vi "MyFPGACode 2.vi"() -> ()   [LabVIEW 2013]
uses:
  <vilib>/Platform/TimedLoop/XDataNode/wakeup.ctl
  <vilib>/Platform/TimedLoop/XDataNode/XDNodeRunTimeDep.lvlib
  <vilib>/Platform/TimedLoop/XDataNode/nitl_modes.ctl
  <vilib>/Platform/TimedLoop/XDataNode/timing_clust.ctl
  <vilib>/Platform/TimedLoop/XDataNode/XDataNode.xnode
  <vilib>/eio/EIONode/EIONode.xnode
  <vilib>/rvi/eio/common/nirviEmuTemplateMethod_errors.vi
  <vilib>/rvi/Analysis/measure/butterworth/XNode/niFpgaButterworthFilter.xnode
  <vilib>/rvi/Analysis/measure/LMRsmpl/XNode/niFPGA Rational Resampler.xnode
  <vilib>/rvi/LocalResourceManager/LocalResourceManager.xnode
  <vilib>/rvi/DataTransferAndStorage/Container/XNode/niFpgaContainer.xnode
  <vilib>/rvi/FIFO/Fifo_Resource/niFpgaFifoEmulationRefIn.vi
  <vilib>/rvi/Analysis/common/codeGenErrors/XNode/niFpgaXNodeCodeGenErrorHandle.vi
  <vilib>/rvi/DataTransferAndStorage/Container/Common/niFpgaContainerGetUniqueNameForEmu.vi
  <vilib>/rvi/DataTransferAndStorage/Container/Common/niFpgaContainerSetEmuInfo.vi
  <vilib>/rvi/eio/common/nirviEmuReportErrorAndStop.vi
panel:
  in  "Start 0":bool
  in  "Filter On":bool=TRUE
  in  "Beta":fxp<+/-,24,0>
  out "Output 8":i16
  out "Output 7":i16
  out "Output 6":i16
  out "Output 5":i16
  out "Output 4":i16
  out "Output 3":i16
  out "Output 2":i16
  out "Output 1":i16
  out "Output 0":i16
  out "Input 8":i16
  out "Input 7":i16
  out "Input 6":i16
  out "Input 5":i16
  out "Input 4":i16
  out "Input 3":i16
  out "Input 2":i16
  out "Input 1":i16
  in  "Local Stop 0":bool
  out "Actual Loop Rate (Ticks)":u32
  out "Late? Latched":bool
  out "Input 0":i16
  in  "Loop Rate (Ticks)":u32=4000
  in  "Reset":bool
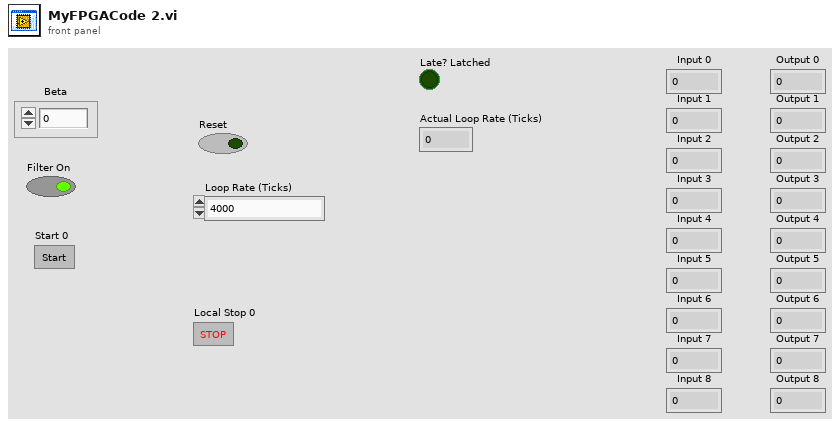
[diagram p1: front panel]
types:
  T1 = typedef "XDNodeRunTimeDep.lvlib/timing_clust.ctl" = cluster{"Expected End [f-1]":u64, "Actual End [f-1]":u64, "Finished Late? [f-1]":bool, "Expected End [i-1]":u64, "Actual End [i-1]":u64, "Finished Late? [i-1]":bool, "Expected Start [i]":u64, "Actual Start [i]":u64, "Expected Start [f]":u64, "Actual Start [f]":u64, "Source Name":string, "Structure Name":string, "Period":i64, "Deadline":i64, "Offset":i64, "Start":i64, "Priority":i32, "Timeout":i32, "Mode":T2, "Wakeup Reason":T3, "Error":errorcluster, "Source Type":string, "Secondary Source Type":string, "Global End Time":u64, "Global Start Time":u64, "Frame Duration":u64, "Iteration Duration":u64, "Assigned CPU":i32, "I/O Scan Engine Mode":u32}
  T2 = typedef "XDNodeRunTimeDep.lvlib/nitl_modes.ctl" = enum32{"No Change", "Process missed periods, maintain original phase", "Discard missed periods, maintain original phase", "Process missed periods, ignore original phase", "Discard missed periods, ignore original phase"}
  T3 = typedef "XDNodeRunTimeDep.lvlib/wakeup.ctl" = enum32{"Normal", "Aborted", "Asynchronous wakeup", "Timing source error", "Timed loop error", "Timeout"}
  T4 = cluster{"X":fxp<+/-,16,2>, "Y":fxp<+/-,16,2>, "Z":fxp<+/-,16,2>}
  T5 = cluster{"[0]":fxp<+/-,16,2>, "[1]":fxp<+/-,16,2>, "[2]":fxp<+/-,16,2>}
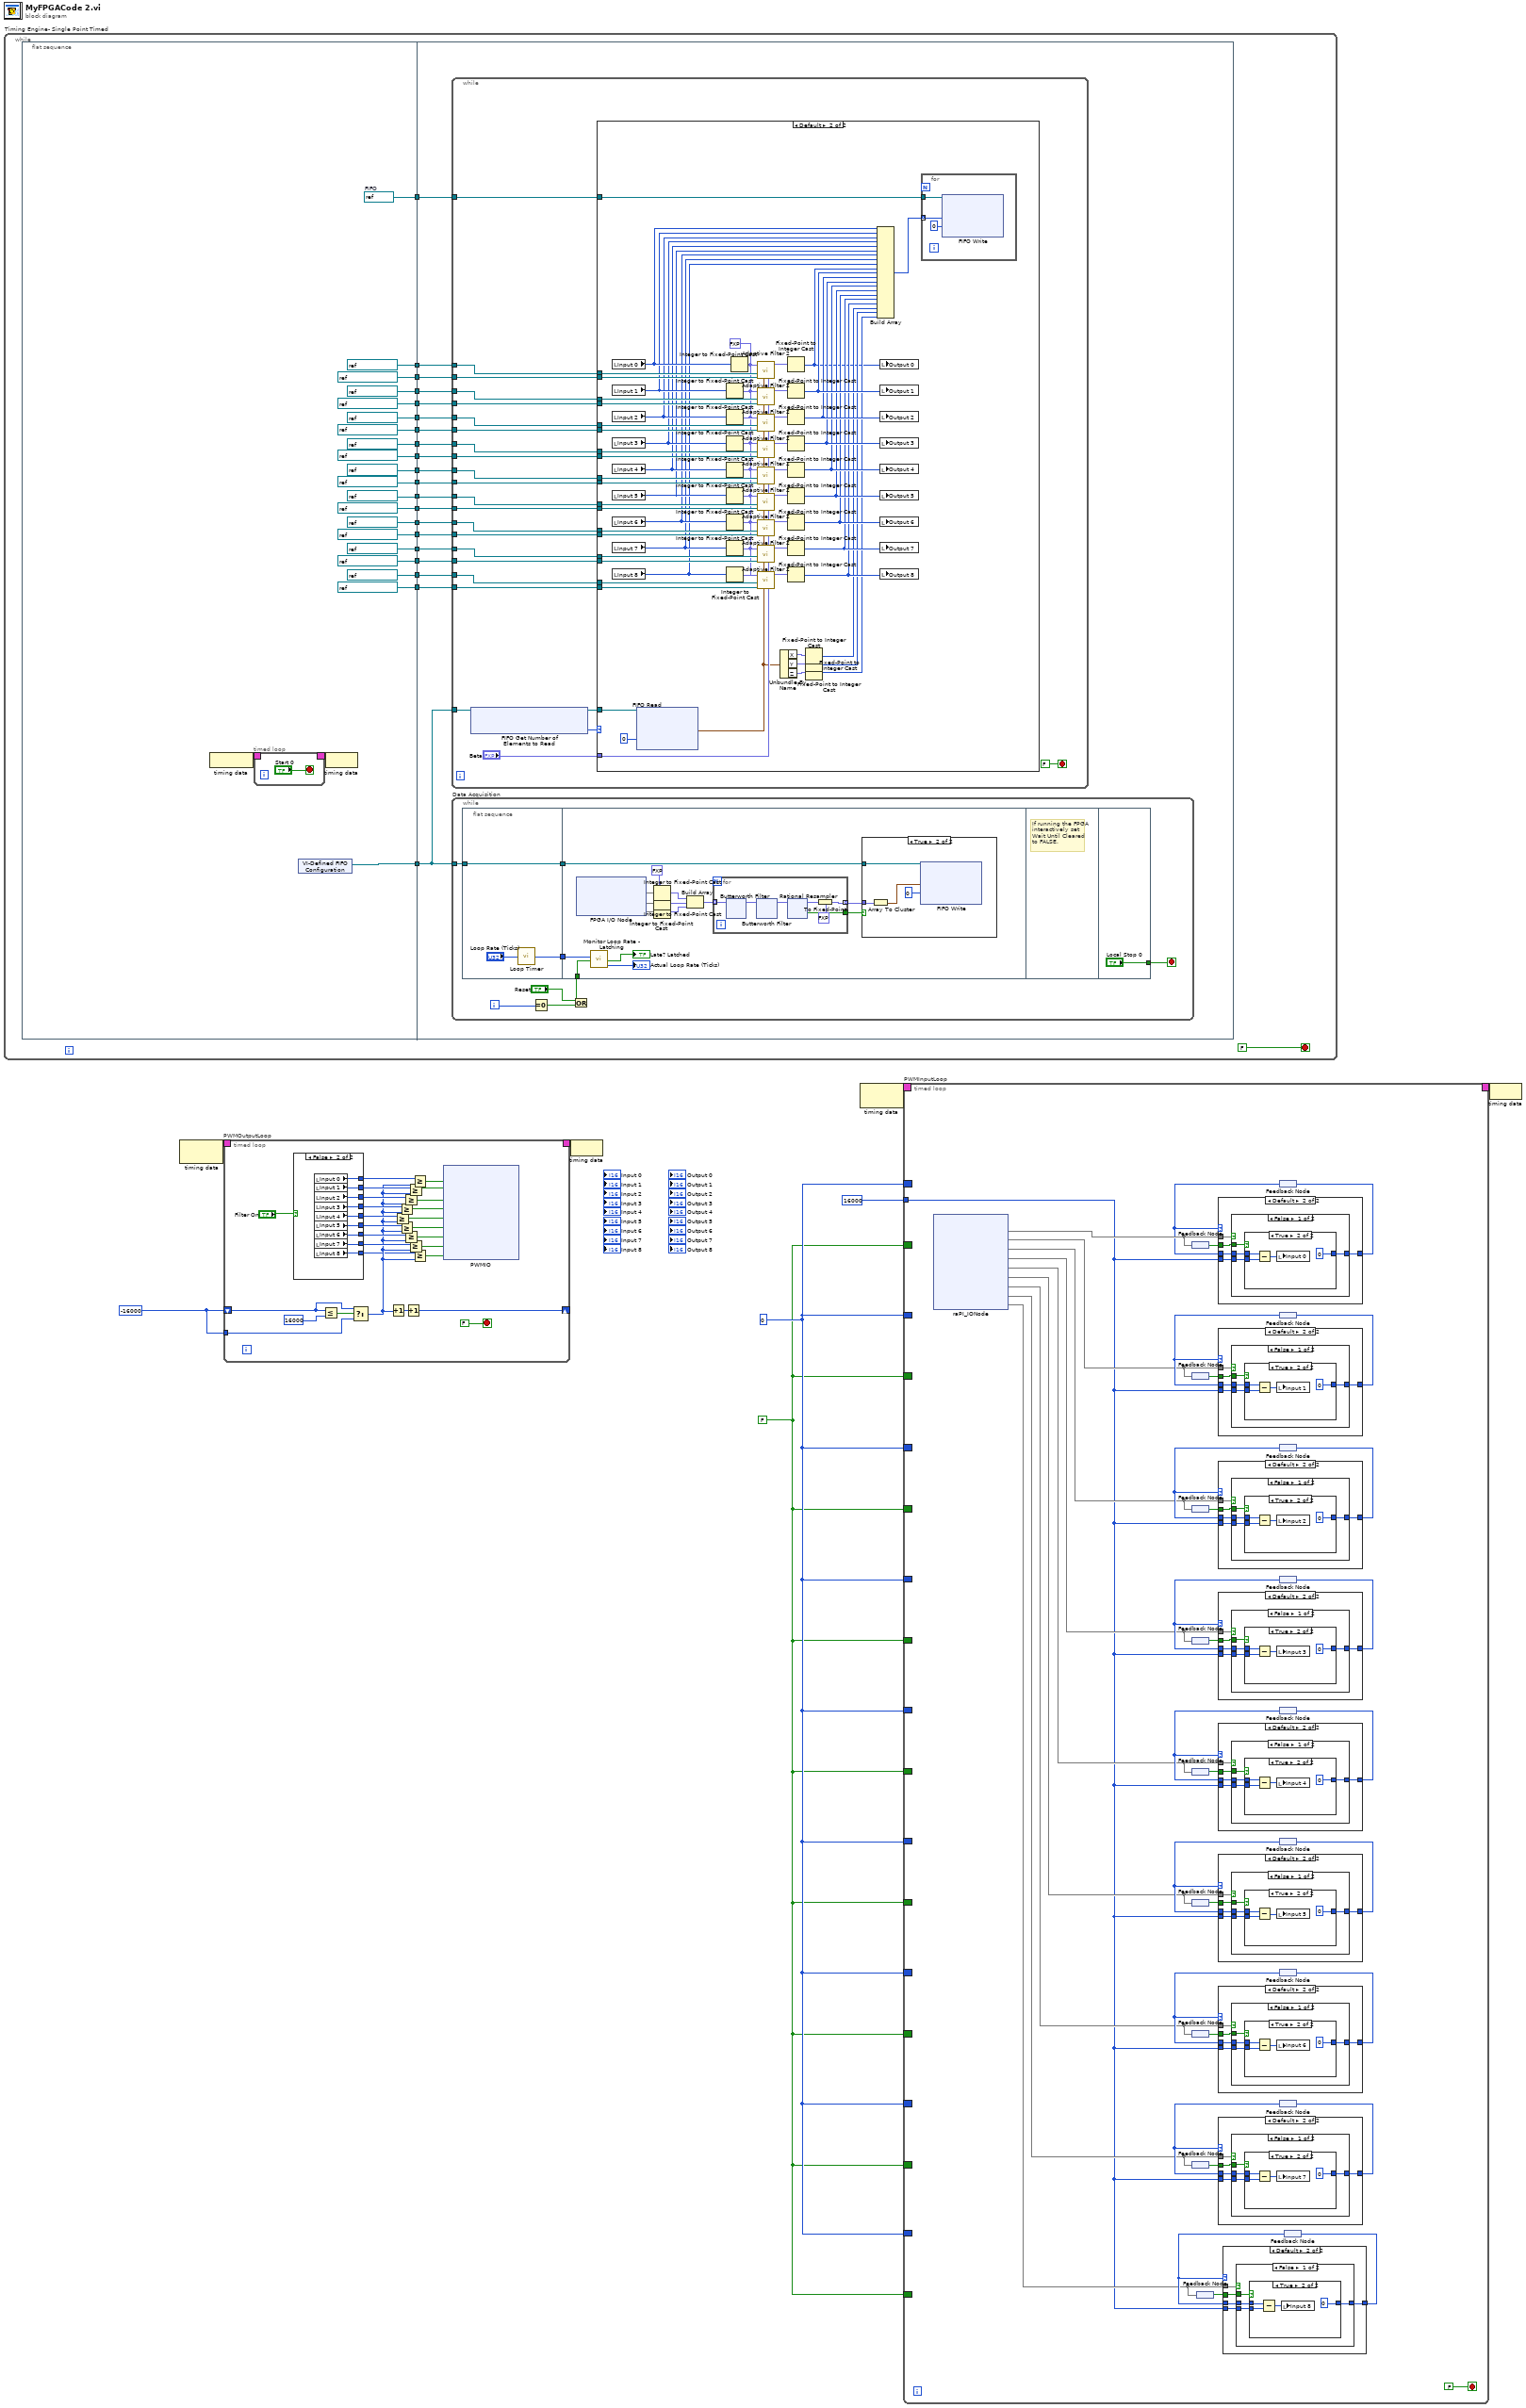
[diagram p0: block diagram]
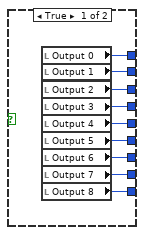
[diagram p2: hidden frame]
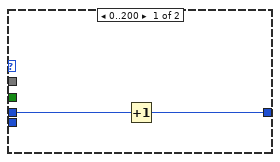
[diagram p3: hidden frame]
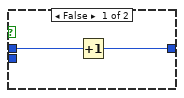
[diagram p4: hidden frame]
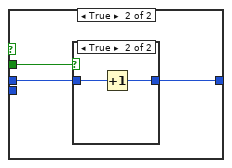
[diagram p5: hidden frame]
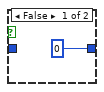
[diagram p6: hidden frame]
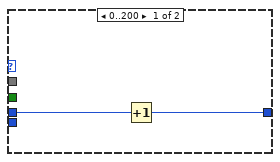
[diagram p7: hidden frame]
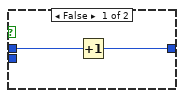
[diagram p8: hidden frame]
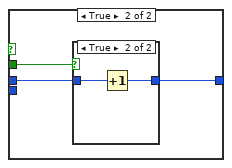
[diagram p9: hidden frame]
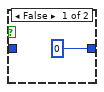
[diagram p10: hidden frame]
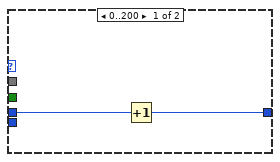
[diagram p11: hidden frame]
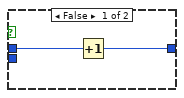
[diagram p12: hidden frame]
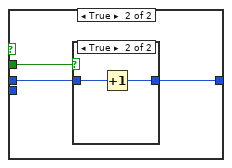
[diagram p13: hidden frame]
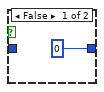
[diagram p14: hidden frame]
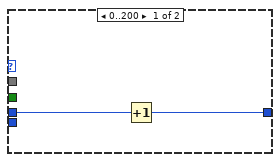
[diagram p15: hidden frame]
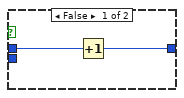
[diagram p16: hidden frame]
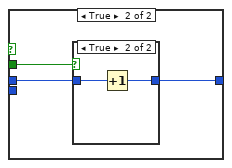
[diagram p17: hidden frame]
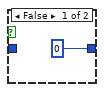
[diagram p18: hidden frame]
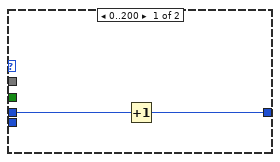
[diagram p19: hidden frame]
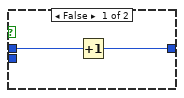
[diagram p20: hidden frame]
diagram:
  w1 = i16 -16000
  w2 = FALSE
  w3 = i16 0
  n1 = while "Timing Engine- Single Point Timed" {
    stop <- FALSE stop-if-true
    n2 = flat-sequence "MainSeq" {
      tunnel: [w51] -> w28
      tunnel: [refnum<k21> "Filter Taps 0" ("Memory")] -> w27
      tunnel: [refnum<k21> "Filter Weights 1" ("Memory")] -> w26
      tunnel: [refnum<k21> "Filter Taps 1" ("Memory")] -> w25
      tunnel: [refnum<k21> "Filter Weights 2" ("Memory")] -> w24
      tunnel: [refnum<k21> "Filter Taps 2" ("Memory")] -> w23
      tunnel: [refnum<k21> "Filter Taps 3" ("Memory")] -> w22
      tunnel: [refnum<k21> "Filter Weights 3" ("Memory")] -> w21
      tunnel: [refnum<k21> "Filter Weights 4" ("Memory")] -> w20
      tunnel: [refnum<k21> "Filter Taps 4" ("Memory")] -> w19
      tunnel: [refnum<k21> "Filter Weights 5" ("Memory")] -> w18
      tunnel: [refnum<k21> "Filter Taps 5" ("Memory")] -> w17
      tunnel: [refnum<k21> "Filter Weights 6" ("Memory")] -> w16
      tunnel: [refnum<k21> "Filter Taps 6" ("Memory")] -> w15
      tunnel: [refnum<k21> "Filter Weights 7" ("Memory")] -> w14
      tunnel: [refnum<k21> "Filter Taps 7" ("Memory")] -> w13
      tunnel: [refnum<k21> "Filter Weights 8" ("Memory")] -> w12
      tunnel: [refnum<k21> "Filter Taps 8" ("Memory")] -> w11
      tunnel: [refnum<k21> "Filter Weights 0" ("Memory")] -> w10
      tunnel: [w30] -> w9
      tunnel: w28 -> [w76]
      tunnel: w27 -> [w75]
      tunnel: w26 -> [w73]
      tunnel: w25 -> [w72]
      tunnel: w24 -> [w71]
      tunnel: w23 -> [w70]
      tunnel: w22 -> [w69]
      tunnel: w21 -> [w68]
      tunnel: w20 -> [w67]
      tunnel: w19 -> [w66]
      tunnel: w18 -> [w65]
      tunnel: w17 -> [w64]
      tunnel: w16 -> [w63]
      tunnel: w15 -> [w62]
      tunnel: w14 -> [w61]
      tunnel: w13 -> [w60]
      tunnel: w12 -> [w59]
      tunnel: w11 -> [w58]
      tunnel: w10 -> [w74]
      tunnel: w9 -> [w57]
      frame #0 {
        w30 = refnum<k21> "FIFO"  # FIFO
        n3 = node-c288 ("Input Node")() -> (w50:T1)
        n4 = timed-loop "initWait" {
          timing: w50 -> [_]
          timing-out: [_] -> w49
          stop <- "Start 0" stop-if-true
        }
        n5 = xnode "VI-Defined FIFO Configuration"() -> ("FIFO Out"=w51:refnum<k21>)
        n6 = node-c288 ("Output Node")(w49) -> ()
      }
      frame #1 {
        n7 = while {
          tunnel: w76 -> [w100]
          tunnel: w75 -> [w96]
          tunnel: w74 -> [w95]
          tunnel: w73 -> [w94]
          tunnel: w72 -> [w93]
          tunnel: w71 -> [w92]
          tunnel: w70 -> [w91]
          tunnel: w69 -> [w90]
          tunnel: w68 -> [w89]
          tunnel: w67 -> [w88]
          tunnel: w66 -> [w87]
          tunnel: w65 -> [w86]
          tunnel: w64 -> [w85]
          tunnel: w63 -> [w84]
          tunnel: w62 -> [w83]
          tunnel: w61 -> [w82]
          tunnel: w60 -> [w81]
          tunnel: w59 -> [w80]
          tunnel: w58 -> [w79]
          tunnel: w57 -> [w77]
          stop <- FALSE stop-if-true
          n8 = xnode ("FIFO Get Number of Elements to Read")("FIFO In"=w100) -> ("Number of Elements to Read"=w99:u32, "FIFO Out"=w98:refnum<k21>)
          n9 = case shown="Default" w99 {
            tunnel: w98 -> [_ w167]
            tunnel: "Beta" -> [_ w125]
            tunnel: w96 -> [_ w164]
            tunnel: w95 -> [_ w139]
            tunnel: w94 -> [_ w141]
            tunnel: w93 -> [_ w162]
            tunnel: w92 -> [_ w160]
            tunnel: w91 -> [_ w159]
            tunnel: w90 -> [_ w158]
            tunnel: w89 -> [_ w157]
            tunnel: w88 -> [_ w156]
            tunnel: w87 -> [_ w155]
            tunnel: w86 -> [_ w154]
            tunnel: w85 -> [_ w153]
            tunnel: w84 -> [_ w152]
            tunnel: w83 -> [_ w151]
            tunnel: w82 -> [_ w150]
            tunnel: w81 -> [_ w149]
            tunnel: w80 -> [_ w148]
            tunnel: w79 -> [_ w147]
            tunnel: w77 -> [_ w103]
            frame 0 {
            }
            frame Default {
              w129 = fxp<+/-,16,2> 0.0 ("fixed-point type")
              n10 = local read "Input 0"() -> (w123:i16)
              n11 = local read "Input 1"() -> (w122:i16)
              n12 = local read "Input 2"() -> (w121:i16)
              n13 = local read "Input 3"() -> (w120:i16)
              n14 = local read "Input 4"() -> (w119:i16)
              n15 = local read "Input 5"() -> (w118:i16)
              n16 = local read "Input 6"() -> (w117:i16)
              n17 = local read "Input 7"() -> (w116:i16)
              n18 = local read "Input 8"() -> (w115:i16)
              n19 = xnode ("FIFO Read")("Timeout"=0, "FIFO In"=w167) -> ("Element"=w124:T4)  [unwired: 2 out]
              n20 = Integer to Fixed-Point Cast(fixed-point type=w129, integer=w122) -> (fixed-point=w137:fxp<+/-,16,2>)
              n21 = Integer to Fixed-Point Cast(fixed-point type=w129, integer=w121) -> (fixed-point=w136:fxp<+/-,16,2>)
              n22 = Integer to Fixed-Point Cast(fixed-point type=w129, integer=w120) -> (fixed-point=w135:fxp<+/-,16,2>)
              n23 = Integer to Fixed-Point Cast(fixed-point type=w129, integer=w119) -> (fixed-point=w134:fxp<+/-,16,2>)
              n24 = Integer to Fixed-Point Cast(fixed-point type=w129, integer=w118) -> (fixed-point=w133:fxp<+/-,16,2>)
              n25 = Integer to Fixed-Point Cast(fixed-point type=w129, integer=w117) -> (fixed-point=w132:fxp<+/-,16,2>)
              n26 = Integer to Fixed-Point Cast(fixed-point type=w129, integer=w116) -> (fixed-point=w131:fxp<+/-,16,2>)
              n27 = Integer to Fixed-Point Cast(fixed-point type=w129, integer=w115) -> (fixed-point=w130:fxp<+/-,16,2>)
              n28 = Integer to Fixed-Point Cast(fixed-point type=w129, integer=w123) -> (fixed-point=w138:fxp<+/-,16,2>)
              n29 = call "Adaptive Filter 2.vi"("Beta"=w125, "Noise"=w124, "Weights"=w139, "Taps"=w164, "Input"=w138) -> ("Error Out"=w165:fxp<+/-,16,2>)  [unwired: 6 in]
              n30 = call "Adaptive Filter 2.vi"("Beta"=w125, "Noise"=w124, "Weights"=w141, "Taps"=w162, "Input"=w137) -> ("Error Out"=w163:fxp<+/-,16,2>)  [unwired: 6 in]
              n31 = call "Adaptive Filter 2.vi"("Beta"=w125, "Noise"=w124, "Weights"=w160, "Taps"=w159, "Input"=w136) -> ("Error Out"=w161:fxp<+/-,16,2>)  [unwired: 6 in]
              n32 = call "Adaptive Filter 2.vi"("Beta"=w125, "Noise"=w124, "Weights"=w157, "Taps"=w158, "Input"=w135) -> ("Error Out"=w146:fxp<+/-,16,2>)  [unwired: 6 in]
              n33 = call "Adaptive Filter 2.vi"("Beta"=w125, "Noise"=w124, "Weights"=w156, "Taps"=w155, "Input"=w134) -> ("Error Out"=w145:fxp<+/-,16,2>)  [unwired: 6 in]
              n34 = call "Adaptive Filter 2.vi"("Beta"=w125, "Noise"=w124, "Weights"=w154, "Taps"=w153, "Input"=w133) -> ("Error Out"=w144:fxp<+/-,16,2>)  [unwired: 6 in]
              n35 = call "Adaptive Filter 2.vi"("Beta"=w125, "Noise"=w124, "Weights"=w152, "Taps"=w151, "Input"=w132) -> ("Error Out"=w143:fxp<+/-,16,2>)  [unwired: 6 in]
              n36 = call "Adaptive Filter 2.vi"("Beta"=w125, "Noise"=w124, "Weights"=w150, "Taps"=w149, "Input"=w131) -> ("Error Out"=w142:fxp<+/-,16,2>)  [unwired: 6 in]
              n37 = call "Adaptive Filter 2.vi"("Beta"=w125, "Noise"=w124, "Weights"=w148, "Taps"=w147, "Input"=w130) -> ("Error Out"=w140:fxp<+/-,16,2>)  [unwired: 6 in]
              n38 = Unbundle By Name(w124) -> ("X"=w128:fxp<+/-,16,2>, "Y"=w127:fxp<+/-,16,2>, "Z"=w126:fxp<+/-,16,2>)
              n39 = Fixed-Point to Integer Cast(1:w165) -> (0:w101:i16)
              n40 = Fixed-Point to Integer Cast(1:w163) -> (0:w114:i16)
              n41 = Fixed-Point to Integer Cast(1:w161) -> (0:w113:i16)
              n42 = Fixed-Point to Integer Cast(1:w146) -> (0:w112:i16)
              n43 = Fixed-Point to Integer Cast(1:w145) -> (0:w111:i16)
              n44 = Fixed-Point to Integer Cast(1:w144) -> (0:w110:i16)
              n45 = Fixed-Point to Integer Cast(1:w143) -> (0:w109:i16)
              n46 = Fixed-Point to Integer Cast(1:w142) -> (0:w108:i16)
              n47 = Fixed-Point to Integer Cast(1:w140) -> (0:w107:i16)
              n48 = Fixed-Point to Integer Cast(1:w128) -> (0:w106:i16)
              n49 = Fixed-Point to Integer Cast(1:w127) -> (0:w105:i16)
              n50 = Fixed-Point to Integer Cast(1:w126) -> (0:w104:i16)
              n51 = Build Array(w123, w122, w121, w120, w119, w118, w117, w116, w115, w101, w114, w113, w112, w111, w110, w109, w108, w107, w106, w105, w104) -> (w102:i16[])
              n52 = local write "Output 0"(w101) -> ()
              n53 = local write "Output 1"(w114) -> ()
              n54 = local write "Output 2"(w113) -> ()
              n55 = local write "Output 3"(w112) -> ()
              n56 = local write "Output 4"(w111) -> ()
              n57 = local write "Output 5"(w110) -> ()
              n58 = local write "Output 6"(w109) -> ()
              n59 = local write "Output 7"(w108) -> ()
              n60 = local write "Output 8"(w107) -> ()
              n61 = for {
                tunnel: w103 -> [w170]
                tunnel: w102 -> [w169] mode=indexing
                n62 = xnode ("FIFO Write")("Element"=w169, "Timeout"=0, "FIFO In"=w170) -> ()  [unwired: 2 out]
              }
            }
          }
        }
        n63 = while "Data Acquisition" {
          tunnel: w76 -> [w173]
          i -> [w171]
          stop <- w178 stop-if-true
          n64 = flat-sequence "Data Acquisition Sequence" {
            tunnel: ["Loop Rate (Ticks)"] -> w177
            tunnel: w173 -> [w180]
            tunnel: [w180] -> w172
            tunnel: w177 -> [w193]
            tunnel: w174 -> [w194]
            tunnel: w172 -> [w190]
            tunnel: ["Local Stop 0"] -> w178
            frame #0 {
              n65 = call "Loop Timer"("Count(Ticks)"="Loop Rate (Ticks)") -> ()  [unwired: 1 out]
            }
            frame #1 {
              w182 = fxp<+/-,16,2> 0.0 ("fixed-point type")
              n66 = xnode "FPGA I/O Node"() -> ("Connector0/AI0"=w183, "Connector0/AI1"=w184, "Connector0/AI2"=w185)  [unwired: 3 in, 3 out]
              n67 = call "Monitor Loop Rate - Latching.vi"("Reset"=w194, "Count(Ticks)"=w193) -> ("Actual Loop Rate (Ticks)"=→"Actual Loop Rate (Ticks)":u32, "Late? (Latched)"=→"Late? Latched":bool)  [unwired: 7 in, 1 out]
              n68 = Integer to Fixed-Point Cast(fixed-point type=w182, integer=w183) -> (fixed-point=w188:fxp<+/-,16,2>)
              n69 = Integer to Fixed-Point Cast(fixed-point type=w182, integer=w184) -> (fixed-point=w187:fxp<+/-,16,2>)
              n70 = Integer to Fixed-Point Cast(fixed-point type=w182, integer=w185) -> (fixed-point=w186:fxp<+/-,16,2>)
              n71 = Build Array(w188, w187, w186) -> (w192:fxp<+/-,16,2>[])
              n72 = for {
                tunnel: w192 -> [w204] mode=indexing
                tunnel: [w201] -> w191 mode=indexing
                tunnel: [w202] -> w189
                n73 = xnode "Butterworth Filter"("input data"=w204) -> ("output data"=w206:fxp<+/-,16,2>)  [unwired: 2 in, 1 out]
                n74 = xnode "Butterworth Filter"("input data"=w206) -> ("output data"=w205:fxp<+/-,16,2>)  [unwired: 2 in, 1 out]
                n75 = xnode "Rational Resampler"("input data"=w205) -> ("output data"=w203:fxp<+/-,18,2>, "output valid"=w202:bool)  [unwired: 1 out]
                n76 = To Fixed-Point(fixed-point type=fxp<+/-,16,2> 0.0, number=w203) -> (fixed-point=w201:fxp<+/-,16,2>)
              }
              n77 = case shown="True" w189 {
                tunnel: w191 -> [_ w199]
                tunnel: w190 -> [_ w198]
                frame False {
                }
                frame True {
                  n78 = Array To Cluster(array=w199) -> (cluster=w197:T5)
                  n79 = xnode ("FIFO Write")("Element"=w197, "Timeout"=0, "FIFO In"=w198) -> ()  [unwired: 2 out]
                }
              }
            }
            frame #2 {
              # "If running the FPGA interactively set Wait Until Cleared to FALSE."
            }
            frame #3 {
            }
          }
          n80 = Equal To 0?(x=w171) -> (x = 0?=w176:bool)
          n81 = Or(x="Reset", y=w176) -> (x .or. y?=w174:bool)
        }
      }
    }
  }
  n82 = node-c288 ("Input Node")() -> (w6:T1)  [unwired: 1 in]
  n83 = timed-loop "PWMOutputLoop" {
    timing: w6 -> [_]
    timing-out: [_] -> w5
    shift-right: [w276] -> _
    shift-left: w1 -> [w299]
    tunnel: w1 -> [w277]
    stop <- FALSE stop-if-true
    n84 = case shown="False" "Filter On" {
      tunnel: [w311 w320] -> w297
      tunnel: [w310 w319] -> w295
      tunnel: [w309 w318] -> w293
      tunnel: [w308 w317] -> w292
      tunnel: [w307 w316] -> w289
      tunnel: [w306 w315] -> w288
      tunnel: [w305 w314] -> w287
      tunnel: [w304 w313] -> w286
      tunnel: [w303 w312] -> w279
      frame True {
        n85 = local read "Output 0"() -> (w311:i16)
        n86 = local read "Output 1"() -> (w310:i16)
        n87 = local read "Output 2"() -> (w308:i16)
        n88 = local read "Output 3"() -> (w309:i16)
        n89 = local read "Output 4"() -> (w304:i16)
        n90 = local read "Output 5"() -> (w305:i16)
        n91 = local read "Output 6"() -> (w307:i16)
        n92 = local read "Output 7"() -> (w306:i16)
        n93 = local read "Output 8"() -> (w303:i16)
      }
      frame False {
        n94 = local read "Input 0"() -> (w320:i16)
        n95 = local read "Input 1"() -> (w319:i16)
        n96 = local read "Input 2"() -> (w317:i16)
        n97 = local read "Input 3"() -> (w318:i16)
        n98 = local read "Input 4"() -> (w313:i16)
        n99 = local read "Input 5"() -> (w314:i16)
        n100 = local read "Input 6"() -> (w316:i16)
        n101 = local read "Input 7"() -> (w315:i16)
        n102 = local read "Input 8"() -> (w312:i16)
      }
    }
    n103 = Less Or Equal?(x=w299, y=i16 16000 ("Period")) -> (x <= y?=w300:bool)
    n104 = Select(t=w299, s=w300, f=w277) -> (s? t:f=w281:i16)
    n105 = Increment(x=w281) -> (x+1=w298:i16)
    n106 = Greater Or Equal?(x=w286, y=w281) -> (x >= y?=w285:bool)
    n107 = Greater Or Equal?(x=w293, y=w281) -> (x >= y?=w290:bool)
    n108 = Greater Or Equal?(x=w287, y=w281) -> (x >= y?=w284:bool)
    n109 = Greater Or Equal?(x=w292, y=w281) -> (x >= y?=w291:bool)
    n110 = Greater Or Equal?(x=w289, y=w281) -> (x >= y?=w283:bool)
    n111 = Increment(x=w298) -> (x+1=w276:i16)
    n112 = Greater Or Equal?(x=w295, y=w281) -> (x >= y?=w294:bool)
    n113 = Greater Or Equal?(x=w288, y=w281) -> (x >= y?=w282:bool)
    n114 = Greater Or Equal?(x=w297, y=w281) -> (x >= y?=w296:bool)
    n115 = Greater Or Equal?(x=w279, y=w281) -> (x >= y?=w280:bool)
    n116 = xnode ("PWMIO")("Connector1/DIO0"=w296, "Connector1/DIO1"=w294, "Connector1/DIO2"=w291, "Connector1/DIO3"=w290, "Connector1/DIO4"=w285, "Connector1/DIO5"=w284, "Connector1/DIO6"=w283, "Connector1/DIO7"=w282, "Connector1/DIO8"=w280) -> ()  [unwired: 9 in, 9 out]
  }
  n117 = node-c288 ("Output Node")(w5) -> ()
  n118 = node-c288 ("Input Node")() -> (w8:T1)  [unwired: 1 in]
  n119 = timed-loop "PWMInputLoop" {
    timing: w8 -> [_]
    timing-out: [_] -> w7
    border: w3 -> [_]
    border: w2 -> [_]
    tunnel: i16 16000 -> [w323]
    border: w3 -> [_]
    border: w2 -> [_]
    border: w3 -> [_]
    border: w2 -> [_]
    border: w3 -> [_]
    border: w2 -> [_]
    border: w3 -> [_]
    border: w2 -> [_]
    border: w3 -> [_]
    border: w2 -> [_]
    border: w3 -> [_]
    border: w2 -> [_]
    border: w3 -> [_]
    border: w2 -> [_]
    border: w3 -> [_]
    border: w2 -> [_]
    stop <- FALSE stop-if-true
    n120 = xnode ("raPI_IONode")() -> ("Connector0/DIO0"=w357, "Connector0/DIO1"=w352, "Connector0/DIO2"=w345, "Connector0/DIO3"=w344, "Connector0/DIO4"=w337, "Connector0/DIO5"=w336, "Connector0/DIO6"=w329, "Connector0/DIO7"=w328, "Connector0/DIO8"=w324)  [unwired: 9 in, 9 out]
    n121 = feedback #1() -> (w358:bool)
    n122 = feedback-in #1(w357) -> ()
    n123 = feedback #2() -> (w354:bool)
    n124 = feedback-in #2(w352) -> ()
    n125 = feedback #3() -> (w347:bool)
    n126 = feedback-in #3(w345) -> ()
    n127 = feedback #4() -> (w350:bool)
    n128 = feedback-in #4(w344) -> ()
    n129 = feedback #5() -> (w342:bool)
    n130 = feedback-in #5(w337) -> ()
    n131 = feedback #6() -> (w339:bool)
    n132 = feedback-in #6(w336) -> ()
    n133 = feedback #7() -> (w331:bool)
    n134 = feedback-in #7(w329) -> ()
    n135 = feedback #8() -> (w334:bool)
    n136 = feedback-in #8(w328) -> ()
    n137 = feedback #9() -> (w326:bool)
    n138 = feedback-in #9(w324) -> ()
    n139 = feedback #10() -> (w356:i16)
    n140 = case shown="Default" w356 {
      tunnel: [w545 w551] -> w359
      tunnel: w356 -> [w546 w550]
      tunnel: w358 -> [_ w549]
      tunnel: w323 -> [_ w548]
      tunnel: w357 -> [_ w547]
      frame 0..200 {
        n141 = Increment(x=w546) -> (x+1=w545:i16)
      }
      frame Default {
        n142 = case shown="False" w547 {
          tunnel: w550 -> [w554 w563]
          tunnel: [w552 w564] -> w551
          tunnel: w549 -> [w555 w562]
          tunnel: w548 -> [w553 _]
          frame False {
            n143 = case shown="True" w555 {
              tunnel: w554 -> [w557 w560]
              tunnel: w553 -> [_ w559]
              tunnel: [w556 i16 0] -> w552
              frame False {
                n144 = Increment(x=w557) -> (x+1=w556:i16)
              }
              frame True {
                n145 = Subtract(x=w560, y=w559) -> (x-y=w561:i16)
                n146 = local write "Input 0"(w561) -> ()
              }
            }
          }
          frame True {
            n147 = case shown="True" w562 {
              tunnel: [i16 0 w567] -> w564
              tunnel: w563 -> [_ w566]
              frame False {
              }
              frame True {
                n148 = Increment(x=w566) -> (x+1=w567:i16)
              }
            }
          }
        }
      }
    }
    n149 = feedback-in #10(w359) -> ()
    n150 = feedback #11() -> (w355:i16)
    n151 = case shown="Default" w355 {
      tunnel: [w522 w528] -> w353
      tunnel: w355 -> [w523 w527]
      tunnel: w354 -> [_ w526]
      tunnel: w323 -> [_ w525]
      tunnel: w352 -> [_ w524]
      frame 0..200 {
        n152 = Increment(x=w523) -> (x+1=w522:i16)
      }
      frame Default {
        n153 = case shown="False" w524 {
          tunnel: w527 -> [w531 w540]
          tunnel: [w529 w541] -> w528
          tunnel: w526 -> [w532 w539]
          tunnel: w525 -> [w530 _]
          frame False {
            n154 = case shown="True" w532 {
              tunnel: w531 -> [w534 w537]
              tunnel: w530 -> [_ w536]
              tunnel: [w533 i16 0] -> w529
              frame False {
                n155 = Increment(x=w534) -> (x+1=w533:i16)
              }
              frame True {
                n156 = Subtract(x=w537, y=w536) -> (x-y=w538:i16)
                n157 = local write "Input 1"(w538) -> ()
              }
            }
          }
          frame True {
            n158 = case shown="True" w539 {
              tunnel: [i16 0 w544] -> w541
              tunnel: w540 -> [_ w543]
              frame False {
              }
              frame True {
                n159 = Increment(x=w543) -> (x+1=w544:i16)
              }
            }
          }
        }
      }
    }
    n160 = feedback-in #11(w353) -> ()
    n161 = feedback #12() -> (w348:i16)
    n162 = case shown="Default" w348 {
      tunnel: [w499 w505] -> w346
      tunnel: w348 -> [w500 w504]
      tunnel: w347 -> [_ w503]
      tunnel: w323 -> [_ w502]
      tunnel: w345 -> [_ w501]
      frame 0..200 {
        n163 = Increment(x=w500) -> (x+1=w499:i16)
      }
      frame Default {
        n164 = case shown="False" w501 {
          tunnel: w504 -> [w508 w517]
          tunnel: [w506 w518] -> w505
          tunnel: w503 -> [w509 w516]
          tunnel: w502 -> [w507 _]
          frame False {
            n165 = case shown="True" w509 {
              tunnel: w508 -> [w511 w514]
              tunnel: w507 -> [_ w513]
              tunnel: [w510 i16 0] -> w506
              frame False {
                n166 = Increment(x=w511) -> (x+1=w510:i16)
              }
              frame True {
                n167 = Subtract(x=w514, y=w513) -> (x-y=w515:i16)
                n168 = local write "Input 2"(w515) -> ()
              }
            }
          }
          frame True {
            n169 = case shown="True" w516 {
              tunnel: [i16 0 w521] -> w518
              tunnel: w517 -> [_ w520]
              frame False {
              }
              frame True {
                n170 = Increment(x=w520) -> (x+1=w521:i16)
              }
            }
          }
        }
      }
    }
    n171 = feedback-in #12(w346) -> ()
    n172 = feedback #13() -> (w349:i16)
    n173 = case shown="Default" w349 {
      tunnel: [w476 w482] -> w351
      tunnel: w349 -> [w477 w481]
      tunnel: w350 -> [_ w480]
      tunnel: w323 -> [_ w479]
      tunnel: w344 -> [_ w478]
      frame 0..200 {
        n174 = Increment(x=w477) -> (x+1=w476:i16)
      }
      frame Default {
        n175 = case shown="False" w478 {
          tunnel: w481 -> [w485 w494]
          tunnel: [w483 w495] -> w482
          tunnel: w480 -> [w486 w493]
          tunnel: w479 -> [w484 _]
          frame False {
            n176 = case shown="True" w486 {
              tunnel: w485 -> [w488 w491]
              tunnel: w484 -> [_ w490]
              tunnel: [w487 i16 0] -> w483
              frame False {
                n177 = Increment(x=w488) -> (x+1=w487:i16)
              }
              frame True {
                n178 = Subtract(x=w491, y=w490) -> (x-y=w492:i16)
                n179 = local write "Input 3"(w492) -> ()
              }
            }
          }
          frame True {
            n180 = case shown="True" w493 {
              tunnel: [i16 0 w498] -> w495
              tunnel: w494 -> [_ w497]
              frame False {
              }
              frame True {
                n181 = Increment(x=w497) -> (x+1=w498:i16)
              }
            }
          }
        }
      }
    }
    n182 = feedback-in #13(w351) -> ()
    n183 = feedback #14() -> (w341:i16)
    n184 = case shown="Default" w341 {
      tunnel: [w453 w459] -> w343
      tunnel: w341 -> [w454 w458]
      tunnel: w342 -> [_ w457]
      tunnel: w323 -> [_ w456]
      tunnel: w337 -> [_ w455]
      frame 0..200 {
        n185 = Increment(x=w454) -> (x+1=w453:i16)
      }
      frame Default {
        n186 = case shown="False" w455 {
          tunnel: w458 -> [w462 w471]
          tunnel: [w460 w472] -> w459
          tunnel: w457 -> [w463 w470]
          tunnel: w456 -> [w461 _]
          frame False {
            n187 = case shown="True" w463 {
              tunnel: w462 -> [w465 w468]
              tunnel: w461 -> [_ w467]
              tunnel: [w464 i16 0] -> w460
              frame False {
                n188 = Increment(x=w465) -> (x+1=w464:i16)
              }
              frame True {
                n189 = Subtract(x=w468, y=w467) -> (x-y=w469:i16)
                n190 = local write "Input 4"(w469) -> ()
              }
            }
          }
          frame True {
            n191 = case shown="True" w470 {
              tunnel: [i16 0 w475] -> w472
              tunnel: w471 -> [_ w474]
              frame False {
              }
              frame True {
                n192 = Increment(x=w474) -> (x+1=w475:i16)
              }
            }
          }
        }
      }
    }
    n193 = feedback-in #14(w343) -> ()
    n194 = feedback #15() -> (w340:i16)
    n195 = case shown="Default" w340 {
      tunnel: [w430 w436] -> w338
      tunnel: w340 -> [w431 w435]
      tunnel: w339 -> [_ w434]
      tunnel: w323 -> [_ w433]
      tunnel: w336 -> [_ w432]
      frame 0..200 {
        n196 = Increment(x=w431) -> (x+1=w430:i16)
      }
      frame Default {
        n197 = case shown="False" w432 {
          tunnel: w435 -> [w439 w448]
          tunnel: [w437 w449] -> w436
          tunnel: w434 -> [w440 w447]
          tunnel: w433 -> [w438 _]
          frame False {
            n198 = case shown="True" w440 {
              tunnel: w439 -> [w442 w445]
              tunnel: w438 -> [_ w444]
              tunnel: [w441 i16 0] -> w437
              frame False {
                n199 = Increment(x=w442) -> (x+1=w441:i16)
              }
              frame True {
                n200 = Subtract(x=w445, y=w444) -> (x-y=w446:i16)
                n201 = local write "Input 5"(w446) -> ()
              }
            }
          }
          frame True {
            n202 = case shown="True" w447 {
              tunnel: [i16 0 w452] -> w449
              tunnel: w448 -> [_ w451]
              frame False {
              }
              frame True {
                n203 = Increment(x=w451) -> (x+1=w452:i16)
              }
            }
          }
        }
      }
    }
    n204 = feedback-in #15(w338) -> ()
    n205 = feedback #16() -> (w332:i16)
    n206 = case shown="Default" w332 {
      tunnel: [w407 w413] -> w330
      tunnel: w332 -> [w408 w412]
      tunnel: w331 -> [_ w411]
      tunnel: w323 -> [_ w410]
      tunnel: w329 -> [_ w409]
      frame 0..200 {
        n207 = Increment(x=w408) -> (x+1=w407:i16)
      }
      frame Default {
        n208 = case shown="False" w409 {
          tunnel: w412 -> [w416 w425]
          tunnel: [w414 w426] -> w413
          tunnel: w411 -> [w417 w424]
          tunnel: w410 -> [w415 _]
          frame False {
            n209 = case shown="True" w417 {
              tunnel: w416 -> [w419 w422]
              tunnel: w415 -> [_ w421]
              tunnel: [w418 i16 0] -> w414
              frame False {
                n210 = Increment(x=w419) -> (x+1=w418:i16)
              }
              frame True {
                n211 = Subtract(x=w422, y=w421) -> (x-y=w423:i16)
                n212 = local write "Input 6"(w423) -> ()
              }
            }
          }
          frame True {
            n213 = case shown="True" w424 {
              tunnel: [i16 0 w429] -> w426
              tunnel: w425 -> [_ w428]
              frame False {
              }
              frame True {
                n214 = Increment(x=w428) -> (x+1=w429:i16)
              }
            }
          }
        }
      }
    }
    n215 = feedback-in #16(w330) -> ()
    n216 = feedback #17() -> (w333:i16)
    n217 = case shown="Default" w333 {
      tunnel: [w384 w390] -> w335
      tunnel: w333 -> [w385 w389]
      tunnel: w334 -> [_ w388]
      tunnel: w323 -> [_ w387]
      tunnel: w328 -> [_ w386]
      frame 0..200 {
        n218 = Increment(x=w385) -> (x+1=w384:i16)
      }
      frame Default {
        n219 = case shown="False" w386 {
          tunnel: w389 -> [w393 w402]
          tunnel: [w391 w403] -> w390
          tunnel: w388 -> [w394 w401]
          tunnel: w387 -> [w392 _]
          frame False {
            n220 = case shown="True" w394 {
              tunnel: w393 -> [w396 w399]
              tunnel: w392 -> [_ w398]
              tunnel: [w395 i16 0] -> w391
              frame False {
                n221 = Increment(x=w396) -> (x+1=w395:i16)
              }
              frame True {
                n222 = Subtract(x=w399, y=w398) -> (x-y=w400:i16)
                n223 = local write "Input 7"(w400) -> ()
              }
            }
          }
          frame True {
            n224 = case shown="True" w401 {
              tunnel: [i16 0 w406] -> w403
              tunnel: w402 -> [_ w405]
              frame False {
              }
              frame True {
                n225 = Increment(x=w405) -> (x+1=w406:i16)
              }
            }
          }
        }
      }
    }
    n226 = feedback-in #17(w335) -> ()
    n227 = feedback #18() -> (w327:i16)
    n228 = case shown="Default" w327 {
      tunnel: [w361 w367] -> w325
      tunnel: w327 -> [w362 w366]
      tunnel: w326 -> [_ w365]
      tunnel: w323 -> [_ w364]
      tunnel: w324 -> [_ w363]
      frame 0..200 {
        n229 = Increment(x=w362) -> (x+1=w361:i16)
      }
      frame Default {
        n230 = case shown="False" w363 {
          tunnel: w366 -> [w370 w379]
          tunnel: [w368 w380] -> w367
          tunnel: w365 -> [w371 w378]
          tunnel: w364 -> [w369 _]
          frame False {
            n231 = case shown="True" w371 {
              tunnel: w370 -> [w373 w376]
              tunnel: w369 -> [_ w375]
              tunnel: [w372 i16 0] -> w368
              frame False {
                n232 = Increment(x=w373) -> (x+1=w372:i16)
              }
              frame True {
                n233 = Subtract(x=w376, y=w375) -> (x-y=w377:i16)
                n234 = local write "Input 8"(w377) -> ()
              }
            }
          }
          frame True {
            n235 = case shown="True" w378 {
              tunnel: [i16 0 w383] -> w380
              tunnel: w379 -> [_ w382]
              frame False {
              }
              frame True {
                n236 = Increment(x=w382) -> (x+1=w383:i16)
              }
            }
          }
        }
      }
    }
    n237 = feedback-in #18(w325) -> ()
  }
  n238 = node-c288 ("Output Node")(w7) -> ()
